vi "swabian_read_stream_buffer.vi"(8 "error in (no error)":errorcluster, 11 "swabian_local_data":T1={"events"={"update_status"=refnum, "update_chart"=refnum, "update_xy"=refnum, "send_channel_data"=refnum}, "stop_q"=refnum, "tagger_reference"=refnum, "connect_button"=refnum, "counter_reference"=refnum, "tagger_stream_reference"=refnum, "log_reference"=refnum, "current_log_offset"=0, "tt20_buffer_q"=refnum, "stream_to_file_button"=refnum, "num_records"=0, "connected?"=FALSE, "plots"=refnum, "histogram_bin_edges"=[], "histogrammer"=refnum, "plot_lifetimes"=refnum, "xy_graph"=refnum, "Reference\nChannel"=enum."ch0", "trigger_channels"=[], "filter_channels"=[], "active_channels"=[], "acq_mode"=0, "Reference\nChannel"=enum."ch0", "acq_time"=0, "leftovers"={"leftover_stamps"=[], "leftover_channels"=[], "any?"=FALSE}, "sync_period_ps"=0, "raw_stream_path"=path "", "Leftovers"={"missing_sync_data"=[], "missing_events"=0}, "first_batch"=0, "first_sync_stamp"=0}) -> (0 "error out":errorcluster, 2 "stop_loop":bool, 3 "swabian_local_data 2":T1={"events"={"update_status"=refnum, "update_chart"=refnum, "update_xy"=refnum, "send_channel_data"=refnum}, "stop_q"=refnum, "tagger_reference"=refnum, "connect_button"=refnum, "counter_reference"=refnum, "tagger_stream_reference"=refnum, "log_reference"=refnum, "current_log_offset"=0, "tt20_buffer_q"=refnum, "stream_to_file_button"=refnum, "num_records"=0, "connected?"=FALSE, "plots"=refnum, "histogram_bin_edges"=[], "histogrammer"=refnum, "plot_lifetimes"=refnum, "xy_graph"=refnum, "Reference\nChannel"=enum."ch0", "trigger_channels"=[], "filter_channels"=[], "active_channels"=[], "acq_mode"=0, "Reference\nChannel"=enum."ch0", "acq_time"=0, "leftovers"={"leftover_stamps"=[], "leftover_channels"=[], "any?"=FALSE}, "sync_period_ps"=0, "raw_stream_path"=path "", "Leftovers"={"missing_sync_data"=[], "missing_events"=0}, "first_batch"=0, "first_sync_stamp"=0})   [LabVIEW 2018]
uses:
  swabian_local_data_tdef.ctl
  swabian_events_tdef.ctl
  update_chart_tdef.ctl
  channel_data_tdef.ctl
  C:/Users/SWIR TCSPC/Desktop/Swabian/lib/TTCSharp32.dll
  lib/TTCSharp32.dll
  swabian_buffer_tdef.ctl
  reference_checkbox_tdef.ctl
  leftovers_struct.ctl
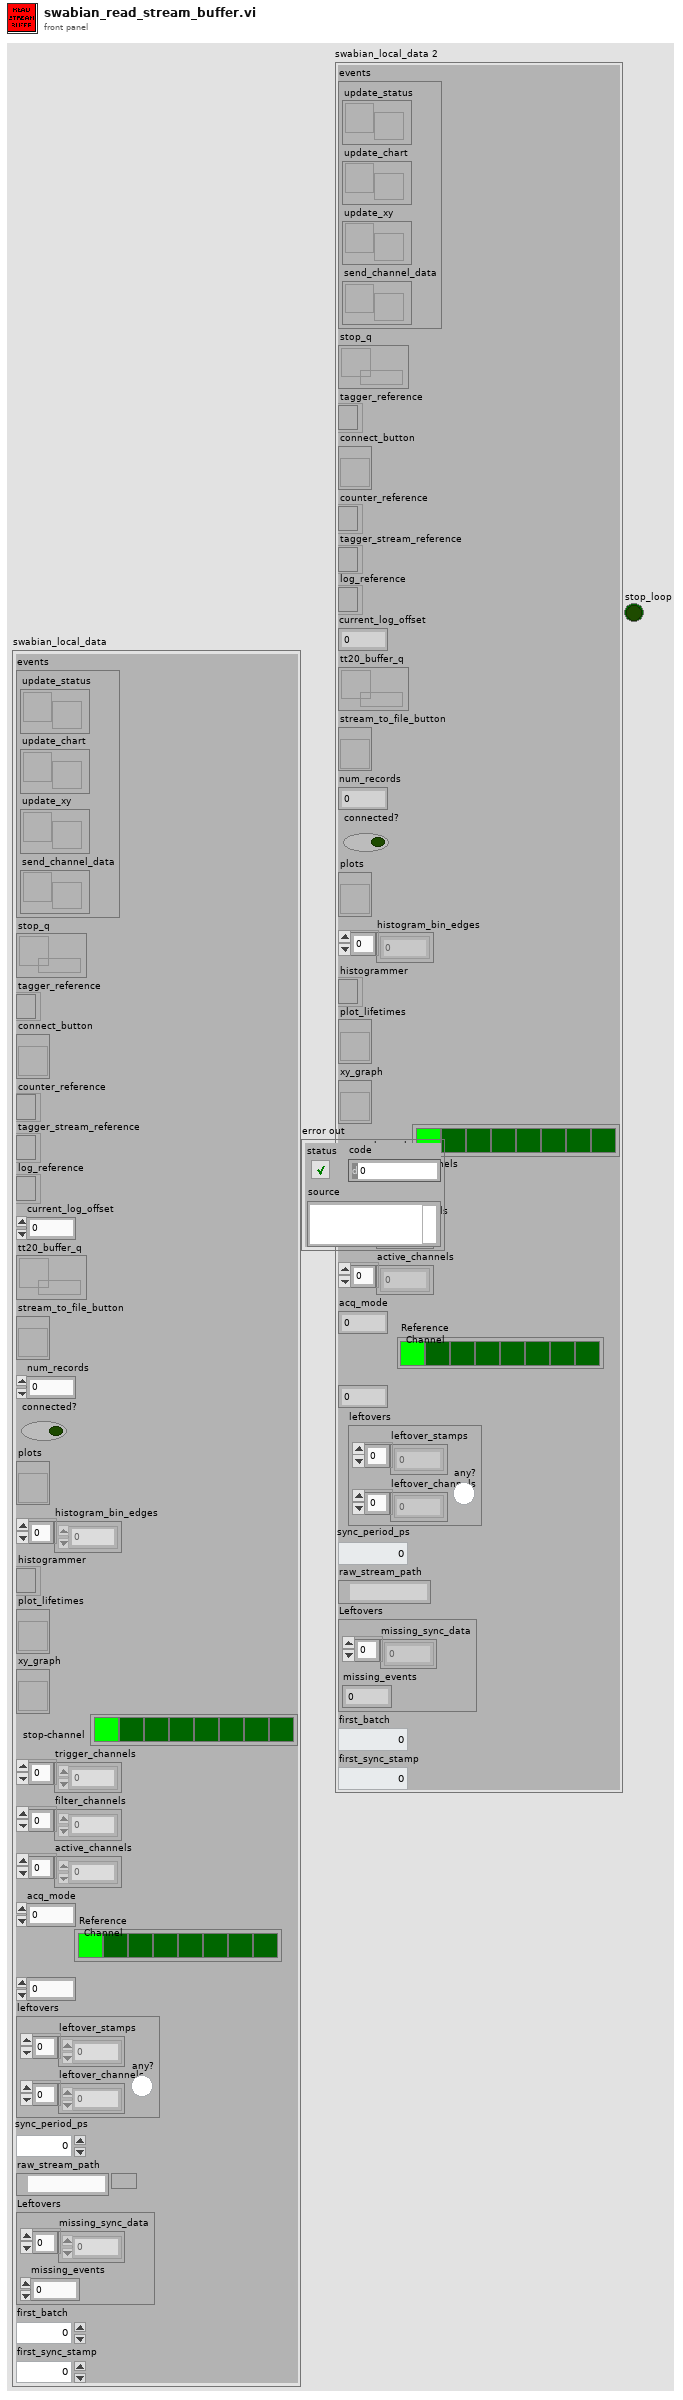
[diagram p1: front panel]
types:
  T1 = typedef "swabian_local_data_tdef.ctl" = cluster{"events":T2, "stop_q":refnum<queue>, "tagger_reference":refnum<k24>, "connect_button":refnum<vi>, "counter_reference":refnum<k24>, "tagger_stream_reference":refnum<k24>, "log_reference":refnum<file>, "current_log_offset":i64, "tt20_buffer_q":refnum<queue>, "stream_to_file_button":refnum<vi>, "num_records":u64, "connected?":bool, "plots":refnum<vi>, "histogram_bin_edges":i64[], "histogrammer":refnum<k24>, "plot_lifetimes":refnum<vi>, "xy_graph":refnum<vi>, "Reference\nChannel":T3, "trigger_channels":i32[], "filter_channels":i32[], "active_channels":i32[], "acq_mode":i32, "Reference\nChannel":T3, "acq_time":i64, "leftovers":T4, "sync_period_ps":i64, "raw_stream_path":path, "Leftovers":cluster{"missing_sync_data":u64[], "missing_events":i32}, "first_batch":i32, "first_sync_stamp":u64}
  T2 = typedef "swabian_events_tdef.ctl" = cluster{"update_status":refnum<user-event>, "update_chart":refnum<user-event>, "update_xy":refnum<user-event>, "send_channel_data":refnum<user-event>}
  T3 = typedef "reference_checkbox_tdef.ctl" = enum32{"No Selection", "ch0", "ch1", "ch2", "ch3", "ch4", "ch5", "ch6", "ch7"}
  T4 = typedef "leftovers_struct.ctl" = cluster{"leftover_stamps":i64[], "leftover_channels":i32[], "any?":bool}
  T5 = typedef "swabian_buffer_tdef.ctl" = cluster{"tagChannels":i32[], "tagTimestamps":i64[], "size":i32}
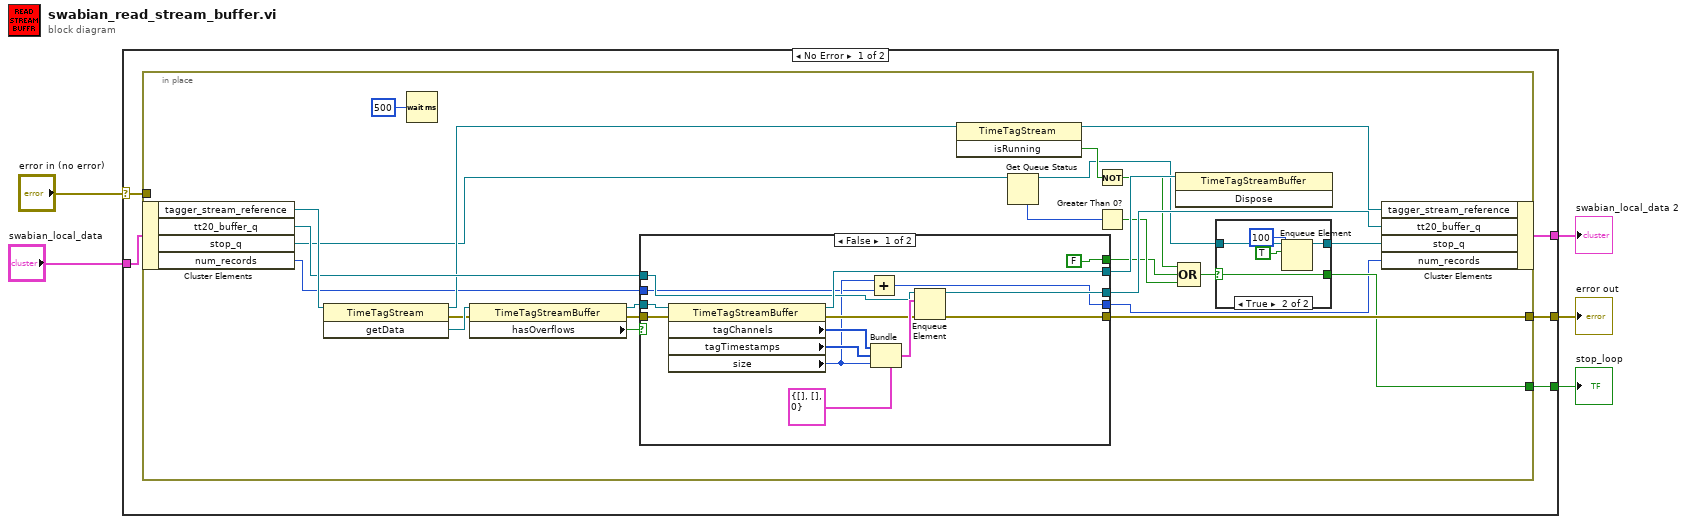
[diagram p0: block diagram]
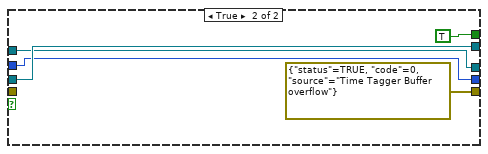
[diagram p3: hidden frame]
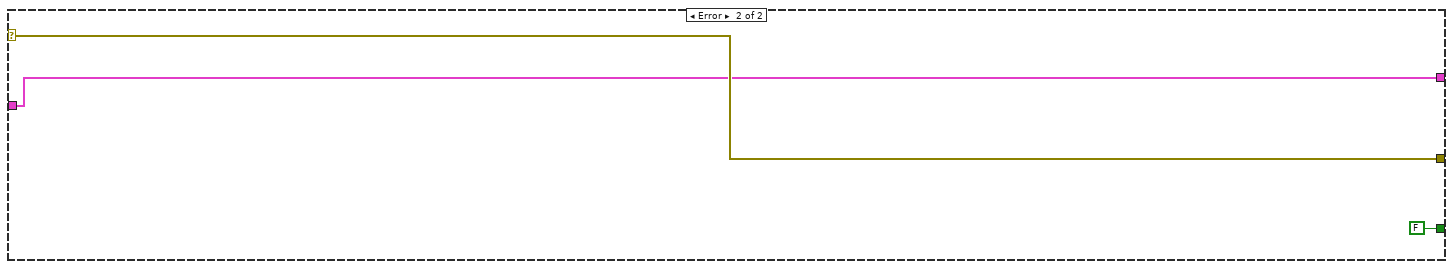
[diagram p4: hidden frame]
diagram:
  n1 = case shown="No Error" "error in (no error)" {
    selector: "error in (no error)" -> [w9 w64]
    tunnel: "swabian_local_data" -> [w10 w63]
    tunnel: [w8 w64] -> w2
    tunnel: [w7 w63] -> w4
    tunnel: [w6 FALSE] -> w1
    frame No Error {
      n2 = in-place {
        in-place-border: w9 -> [_]
        in-place-border: [w24] -> w8
        in-place-border: [w19] -> w6
        n3 = in-place-cluster #1(w10) -> ("tagger_stream_reference"=w35:refnum<k24>, "tt20_buffer_q"=w28:refnum<queue>, "stop_q"=w21:refnum<queue>, "num_records"=w16:u64)
        n4 = invoke class="TimeTagStream" method="getData"(reference=w35) -> (reference out=w26:refnum<k24>, error out=w31:errorcluster, "getData"=w34:refnum<k24>)  [unwired: 2 in]
        n5 = Wait (ms)(milliseconds to wait=u32 500) -> ()  [unwired: 1 out]
        n6 = property class="TimeTagStreamBuffer"(reference=w34, error in=w31) -> (reference out=w33:refnum<k24>, error out=w29:errorcluster, "hasOverflows"=w32:bool)
        n7 = case shown="False" w32 {
          tunnel: w33 -> [w57 w62]
          tunnel: [w56 w62] -> w30
          tunnel: w29 -> [w55 _]
          tunnel: [w47 errorcluster {"status"=TRUE, "code"=0, "source"="Time Tagger Buffer overflow"} ("error out")] -> w24
          tunnel: [FALSE TRUE] -> w13
          tunnel: w28 -> [w50 w59]
          tunnel: [w49 w59] -> w27
          tunnel: w16 -> [w44 w58]
          tunnel: [w43 w58] -> w15
          frame False {
            n8 = property class="TimeTagStreamBuffer"(reference=w57, error in=w55) -> (reference out=w56:refnum<k24>, error out=w48:errorcluster, "tagChannels"=w53:i32[], "tagTimestamps"=w52:i64[], "size"=w45:i32)
            n9 = Add(x=w45, y=w44) -> (x+y=w43:u64)
            n10 = Bundle(cluster=T5 {"tagChannels"=[], "tagTimestamps"=[], "size"=0} ("swabian_buffer"), "tagChannels"=w53, "tagTimestamps"=w52, "size"=w45) -> (w51:T5)
            n11 = Enqueue Element(queue=w50, element=w51, error in (no error)=w48) -> (queue out=w49:refnum<queue>, error out=w47:errorcluster)  [unwired: 1 in, 1 out]
          }
          frame True {
          }
        }
        n12 = invoke class="TimeTagStream" method="isRunning"(reference=w26) -> (reference out=w25:refnum<k24>, "isRunning"=w23:bool)  [unwired: 2 in, 1 out]
        n13 = Get Queue Status(queue=w21) -> (queue out=w18:refnum<queue>, # elements in queue=w20:i32)  [unwired: 2 in, 6 out]
        n14 = Not(x=w23) -> (.not. x?=w12:bool)
        n15 = Greater Than 0?(x=w20) -> (x > 0?=w14:bool)
        n16 = invoke class="TimeTagStreamBuffer" method="Dispose"(reference=w30) -> ()  [unwired: 2 in, 3 out]
        n17 = Compound Arithmetic op=OR(w12, w13, w14) -> (w11:bool)
        n18 = case shown="True" w11 {
          selector: w11 -> [w37 w41]
          tunnel: [w37 w41] -> w19
          tunnel: w18 -> [w36 w40]
          tunnel: [w36 w39] -> w17
          frame False {
          }
          frame True {
            n19 = Enqueue Element(queue=w40, element=TRUE, timeout in ms (-1)=100) -> (queue out=w39:refnum<queue>)  [unwired: 1 in, 2 out]
          }
        }
        n20 = in-place-cluster #1("tagger_stream_reference"=w25, "tt20_buffer_q"=w27, "stop_q"=w17, "num_records"=w15) -> (w7:T1)
      }
    }
    frame Error {
    }
  }
  "swabian_local_data 2" <- w4
  "error out" <- w2
  "stop_loop" <- w1
